vi "AlliGator Fit Termination Criteria & Quality Metrics Output String.vi"(8 "Error In":errorcluster, 9 "Fit Output":T4, 11 "Termination Criteria":T1) -> (0 "Error Out":errorcluster, 1 "Weighted Fit":bool, 3 "String":string)   [LabVIEW 2021, in "AlliGator Decay Analysis.lvlib" / "AlliGator Decay Fit.lvlib"]
doc: "Creates a string describing the fit termination criteria and quality metrics."
uses:
  AlliGator Decay Fit.lvlib
  Fits/Non-linear Fit Output v3.ctl
  Fits/Nonlinear Fit Method.ctl
  <vilib>/Analysis/Matrix/Datatypes/RealMatrix.ctl
  Fits/Convergence Criteria.ctl
  Fits/Non-linear Fitting Algorithm.ctl
  Graphs/XY Graph/XY Plot Data.ctl
  Fits/Fits.lvlib
  <vilib>/Analysis/Matrix/NI_Matrix.lvlib
  Graphs/XY Graph/XY Graph Add-Ons.lvlib
panel:
  in  "Fitting Method":T2
  in  "Fitting Algorithm":T3
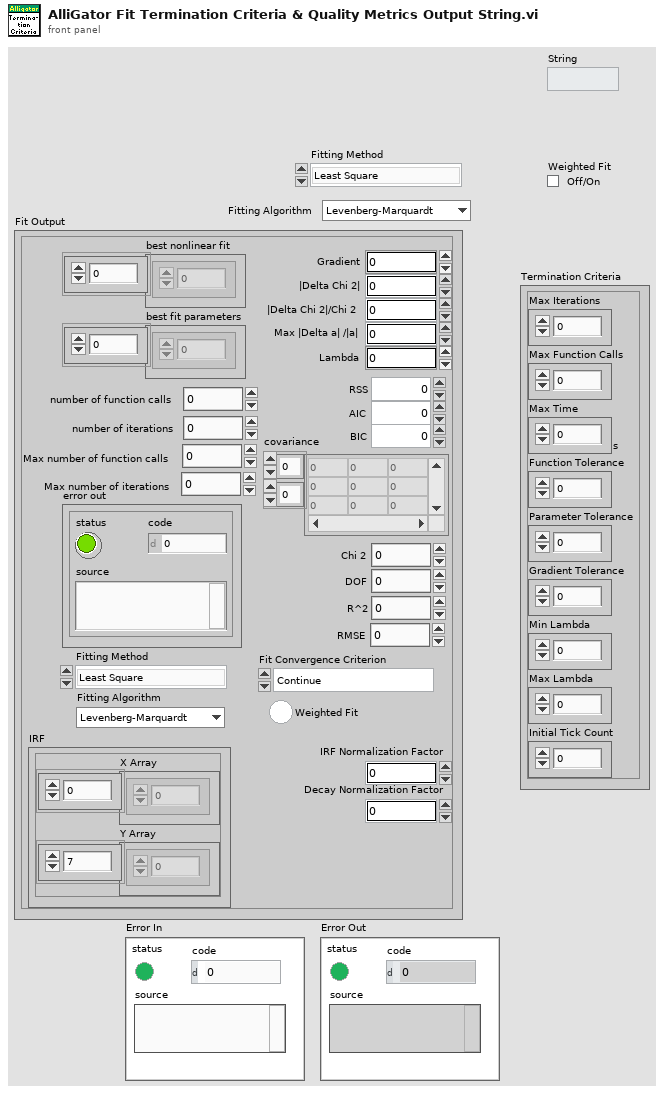
[diagram p1: front panel]
types:
  T1 = cluster{"Max Iterations":i32, "Max Function Calls":i32, "Max Time":dbl[unit], "Function Tolerance":dbl, "Parameter Tolerance":dbl, "Gradient Tolerance":dbl, "Min Lambda":dbl, "Max Lambda":dbl, "Initial Tick Count":u32}
  T2 = typedef "Fits.lvlib/Nonlinear Fit Method.ctl" = enum16{"Least Square", "Least Absolute Residual", "Bisquare", "MLE"}
  T3 = typedef "Fits.lvlib/Non-linear Fitting Algorithm.ctl" = enum16{"Levenberg-Marquardt", "Trust-Region Dogleg"}
  T4 = typedef "Fits.lvlib/Non-linear Fit Output v3.ctl" = cluster{"best nonlinear fit":dbl[], "best fit parameters":dbl[], "R^2":dbl, "RMSE":dbl, "error out":errorcluster, "Fitting Method":T2, "number of function calls":i32, "number of iterations":i32, "covariance":T5, "Chi 2":dbl, "DOF":i32, "Fit Convergence Criterion":T6, "Fitting Algorithm":T3, "Weighted Fit":bool, "Gradient":dbl, "|Delta Chi 2|":dbl, "|Delta Chi 2|/Chi 2":dbl, "Max |Delta a| /|a|":dbl, "Lambda":dbl, "RSS":dbl, "AIC":dbl, "BIC":dbl, "Max number of function calls":i32, "Max number of iterations":i32, "IRF":T7, "IRF Normalization Factor":dbl, "Decay Normalization Factor":dbl}
  T5 = typedef "NI_Matrix.lvlib/RealMatrix.ctl" = dbl[][]
  T6 = typedef "Fits.lvlib/Convergence Criteria.ctl" = enum16{"Continue", "Tolerances Exceeded", "Max Time Exceeded", "Max Iterations Exceeded", "Max Function Evaluations Exceeded", "Scale Range Exceeded"}
  T7 = typedef "XY Graph Add-Ons.lvlib/XY Plot Data.ctl" = cluster{"X Array":dbl[], "Y Array":dbl[]}
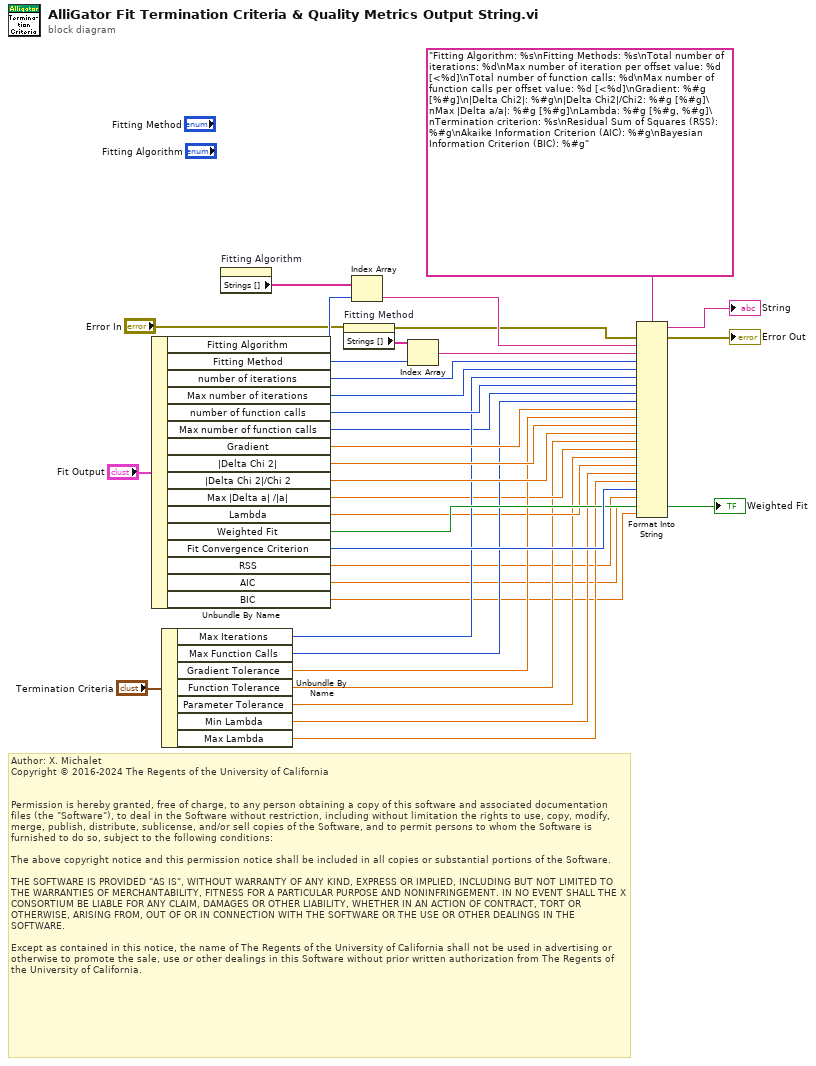
[diagram p0: block diagram]
diagram:
  # "Author: X. Michalet\nCopyright © 2016-2024 The Regents of the University of California\n \n\nPermission is hereby granted, free of charge, to any person obtaining a copy of this software and associated documentation files (the \"Software\"), to deal in the Software without restriction, including without limitation the rights to use, copy, modify, merge, publish, distribute, sublicense, and/or sell copies of the Software, and to permit persons to whom the Software is furnished to do so, subject to the following conditions:\n\nThe above copyright notice and this permission notice shall be included in all copies or substantial portions of the Software.\n\nTHE SOFTWARE IS PROVIDED \"AS IS\", WITHOUT WARRANTY OF ANY KIND, EXPRESS OR IMPLIED, INCLUDING BUT NOT LIMITED TO THE WARRANTIES OF MERCHANTABILITY, FITNESS FOR A PARTICULAR PURPOSE AND NONINFRINGEMENT. IN NO EVENT SHALL THE X CONSORTIUM BE LIABLE FOR ANY CLAIM, DAMAGES OR OTHER LIABILITY, WHETHER IN AN ACTION OF CONTRACT, TORT OR OTHERWISE, ARISING FROM, OUT OF OR IN CONNECTION WITH THE SOFTWARE OR THE USE OR OTHER DEALINGS IN THE SOFTWARE.\n\nExcept as contained in this notice, the name of The Regents of the University of California shall not be used in advertising or otherwise to promote the sale, use or other dealings in this Software without prior written authorization from The Regents of the University of California."
  n1 = Unbundle By Name("Fit Output") -> ("Fitting Algorithm"=w31:T3, "Fitting Method"=w25:T2, "number of iterations"=w26:i32, "Max number of iterations"=w2:i32, "number of function calls"=w27:i32, "Max number of function calls"=w1:i32, "Gradient"=w21:dbl, "|Delta Chi 2|"=w20:dbl, "|Delta Chi 2|/Chi 2"=w19:dbl, "Max |Delta a| /|a|"=w11:dbl, "Lambda"=w10:dbl, "Weighted Fit"=→"Weighted Fit":bool, "Fit Convergence Criterion"=w34:T6, "RSS"=w5:dbl, "AIC"=w4:dbl, "BIC"=w3:dbl)
  n2 = Unbundle By Name("Termination Criteria") -> ("Max Iterations"=w14:i32, "Max Function Calls"=w13:i32, "Gradient Tolerance"=w12:dbl, "Function Tolerance"=w9:dbl, "Parameter Tolerance"=w8:dbl, "Min Lambda"=w7:dbl, "Max Lambda"=w6:dbl)
  n3 = property on="Fitting Algorithm" class="Enum (strict)"() -> ("Strings []"=w22:string[])  [unwired: 2 in, 2 out]
  n4 = property on="Fitting Method" class="Enum (strict)"(error in="Error In") -> (error out=w17:errorcluster, "Strings []"=w23:string[])  [unwired: 1 in, 1 out]
  n5 = Index Array(array=w22, index=w31) -> (element=w32:string)
  n6 = Index Array(array=w23, index=w25) -> (element=w30:string)
  n7 = Format Into String(format string="Fitting Algorithm: %s\nFitting Methods: %s\nTotal number of iterations: %d\nMax number of iteration per offset value: %d [<%d]\nTotal number of function calls: %d\nMax number of function calls per offset value: %d [<%d]\nGradient: %#g [%#g]\n|Delta Chi2|: %#g\n|Delta Chi2|/Chi2: %#g [%#g]\nMax |Delta a/a|: %#g [%#g]\nLambda: %#g [%#g, %#g]\nTermination criterion: %s\nResidual Sum of Squares (RSS): %#g\nAkaike Information Criterion (AIC): %#g\nBayesian Information Criterion (BIC): %#g", error in=w17, w32, w30, w26, w2, w14, w27, w1, w13, w21, w12, w20, w19, w9, w11, w8, w10, w7, w6, w34, w5, w4, w3) -> (resulting string=→"String":string, error out=→"Error Out":errorcluster)  [unwired: 1 in]
